vi "Entry Initialize (User).vi"(8 "error in":errorcluster, 11 "Node in":refnum<class "AMS Cycler Template.lvclass">) -> (0 "error out":errorcluster, 3 "Node out":refnum<class "AMS Cycler Template.lvclass">)   [LabVIEW 2023, in "AMS Cycler Template.lvlib" / "AMS Cycler Template.lvclass"]
uses:
  AMS Cycler Template.lvclass
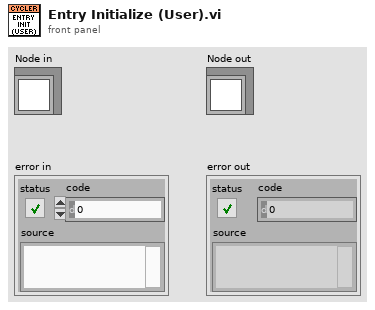
[diagram p1: front panel]
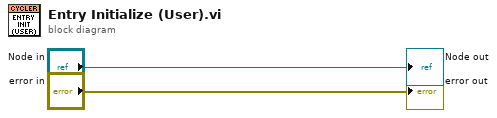
[diagram p0: block diagram]
diagram:
  "Node out" <- "Node in"
  "error out" <- "error in"
